vi "test_pid_amplitude.vi"() -> ()   [LabVIEW 2013]
panel:
  out "Waveform Graph 6":dbl[][](graph)
  out "Waveform Graph 5":dbl[](graph)
  in  "Kp":fxp<+/-,32,6>=0.004999995231628418
  in  "Kd/Tau":fxp<+/-,32,6>
  in  "Ki*Tau":fxp<+/-,32,6>=4.999339580535889e-05
  out "Waveform Graph 4":dbl[](graph)
  out "Waveform Graph 3":dbl[](graph)
  out "Waveform Graph 2":dbl[][](graph)
  out "size(s)":i32[](array[numeric])
  out "Waveform Graph":dbl[][](graph)
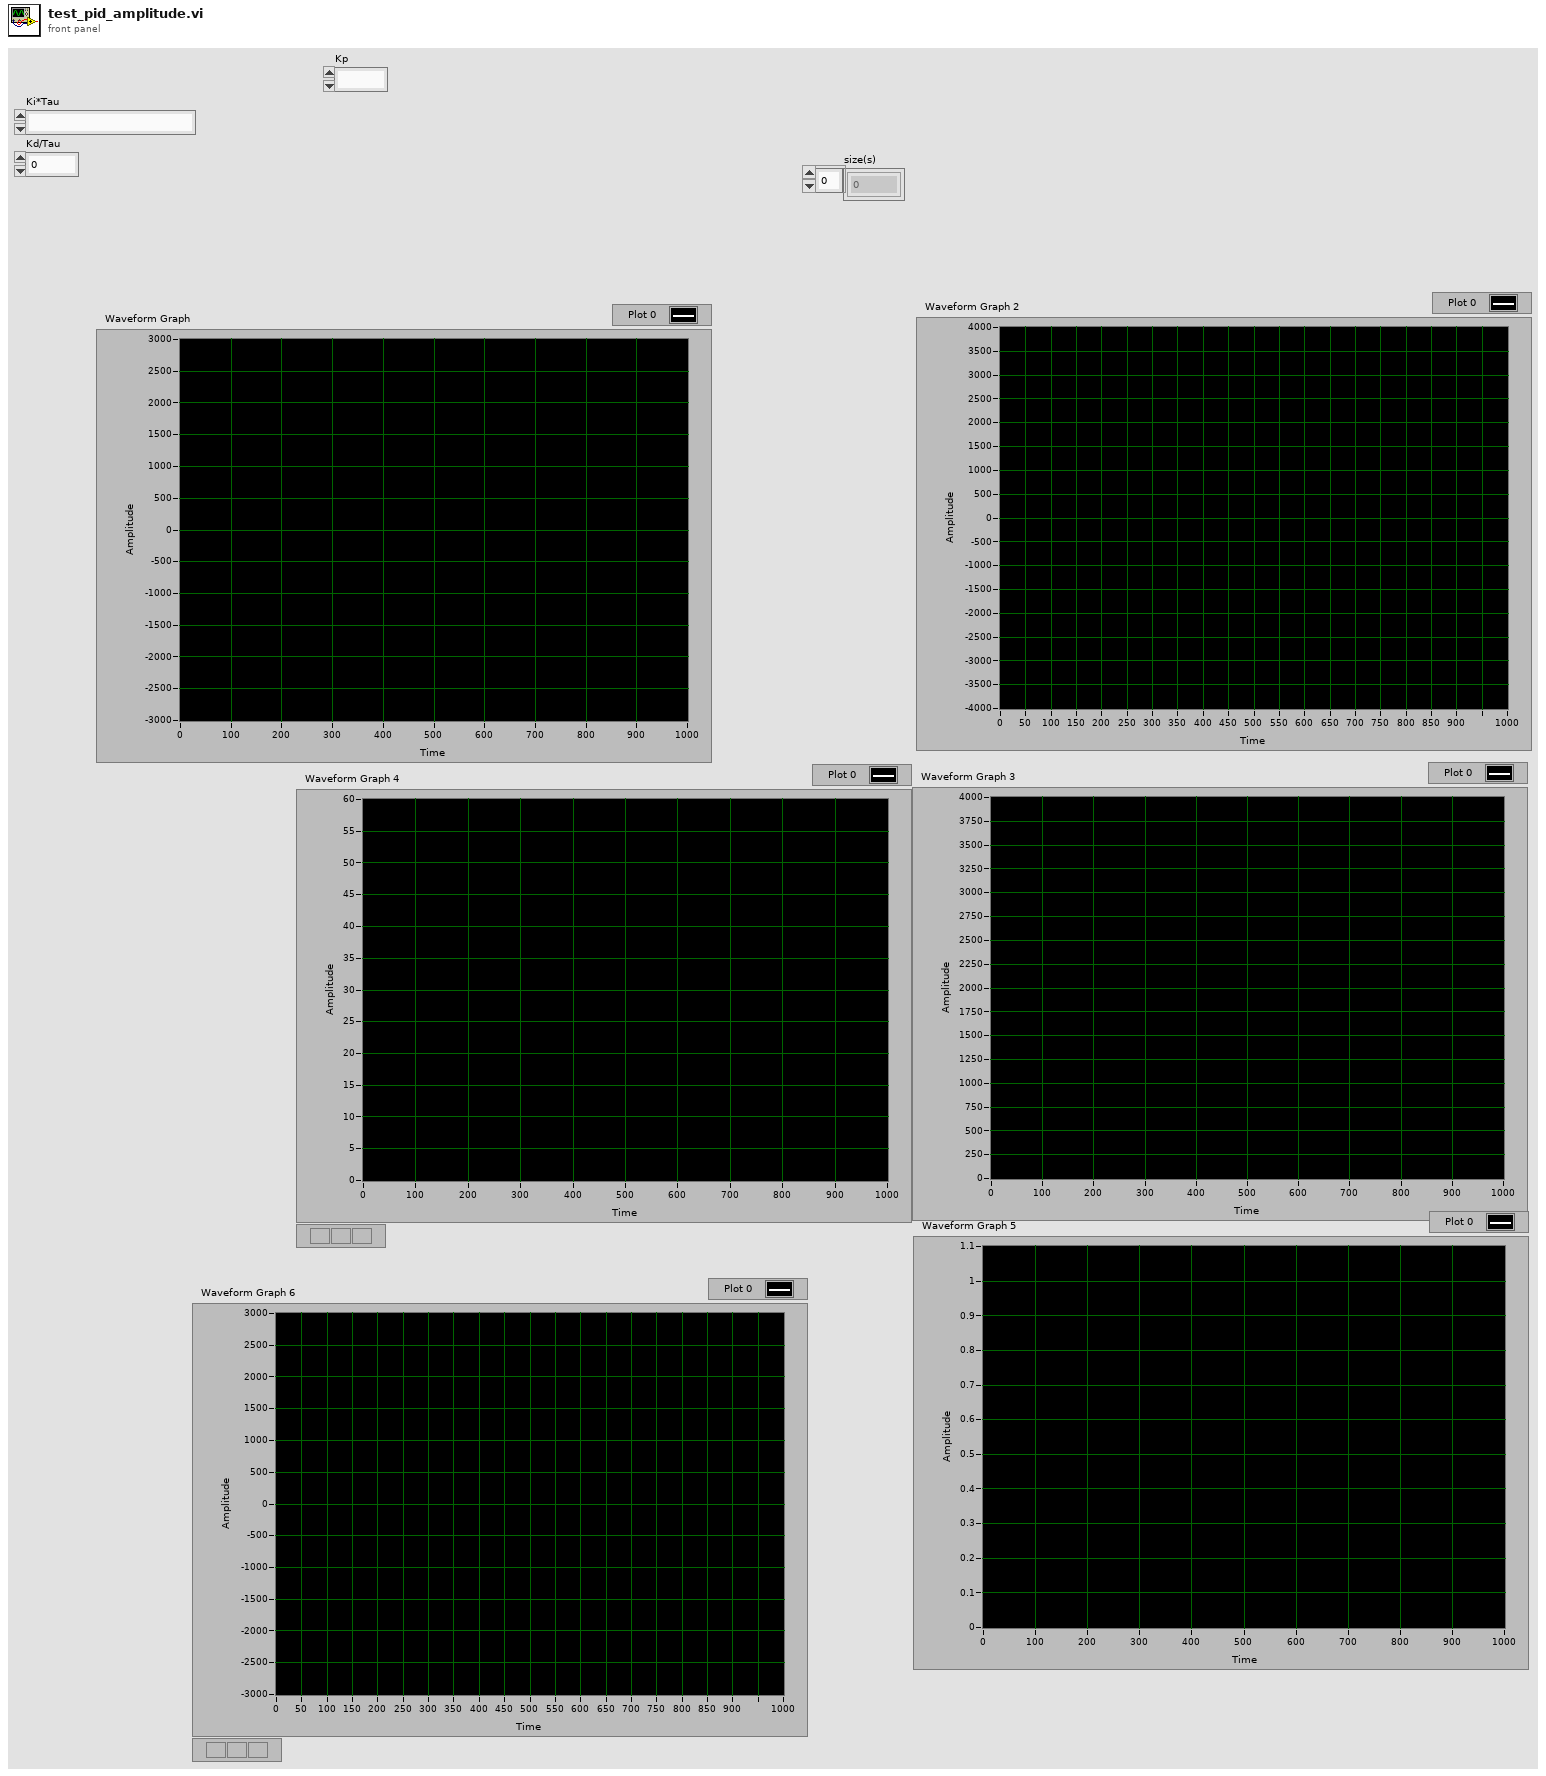
[diagram p1: front panel]
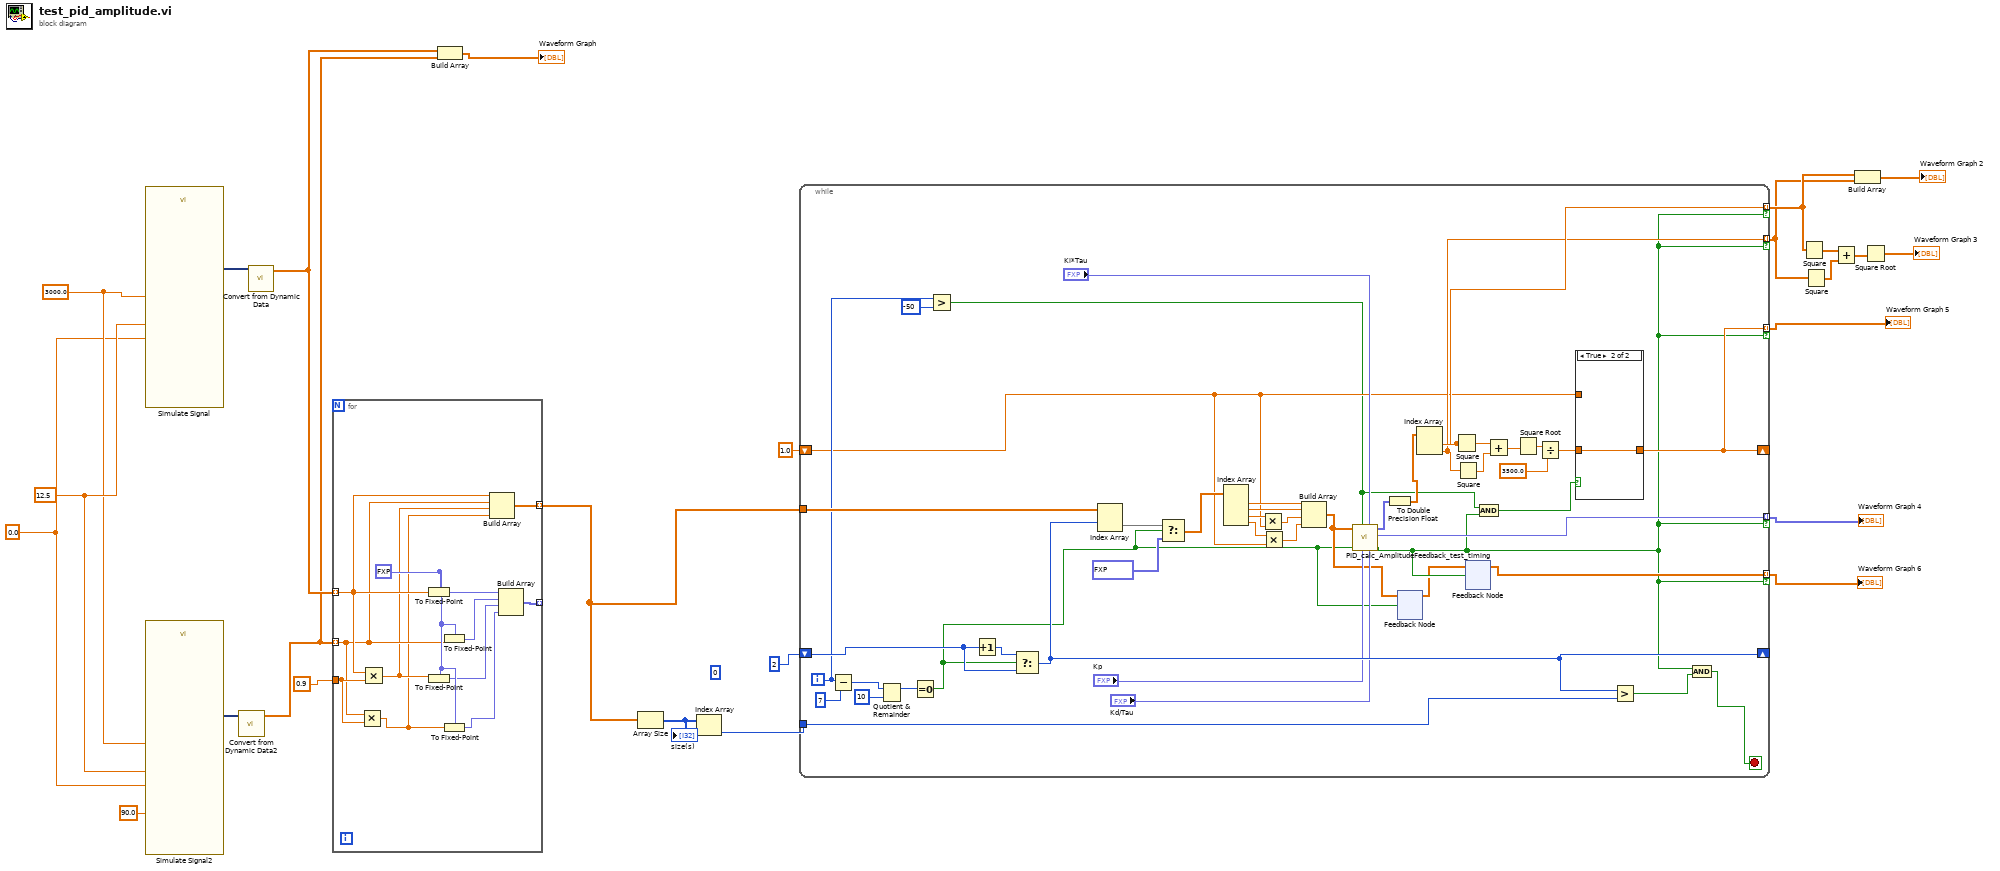
[diagram p0: block diagram]
diagram:
  w12 = 3000.0 ("Amplitude")
  (unwired) 0
  w13 = 12.5 ("Frequency")
  w5 = 0.0 ("Noise amplitude")
  n1 = call "Simulate Signal"("Frequency"=w13, "Amplitude"=w12, "Noise amplitude"=w5) -> ("Sine with Uniform Noise"=w25:dynamicdata)  [unwired: 11 in, 1 out]
  n2 = call "Simulate Signal2"("Frequency"=w13, "Amplitude"=w12, "Phase"=90.0, "Noise amplitude"=w5) -> ("Sine with Uniform Noise"=w23:dynamicdata)  [unwired: 10 in, 1 out]
  n3 = call "Convert from Dynamic Data2"("Dynamic Data Type"=w23) -> ("Array"=w21:dbl[])  [unwired: 3 in]
  n4 = call "Convert from Dynamic Data"("Dynamic Data Type"=w25) -> ("Array"=w22:dbl[])  [unwired: 3 in]
  n5 = for {
    tunnel: w21 -> [w29] mode=indexing
    tunnel: w22 -> [w30] mode=indexing
    tunnel: [w35] -> _ mode=indexing
    tunnel: 0.9 ("y") -> [w34]
    tunnel: [w26] -> w3 mode=indexing
    w33 = fxp<+/-,16,14> 0.0 ("f")
    n6 = Multiply(x=w29, y=w34) -> (x*y=w27:dbl)
    n7 = Multiply(x=w30, y=w34) -> (x*y=w28:dbl)
    n8 = To Fixed-Point(fixed-point type=w33, number=w30) -> (fixed-point=w37:fxp<+/-,16,14>)
    n9 = To Fixed-Point(fixed-point type=w33, number=w28) -> (fixed-point=w31:fxp<+/-,16,14>)
    n10 = To Fixed-Point(fixed-point type=w33, number=w29) -> (fixed-point=w36:fxp<+/-,16,14>)
    n11 = To Fixed-Point(fixed-point type=w33, number=w27) -> (fixed-point=w32:fxp<+/-,16,14>)
    n12 = Build Array(w30, w29, w28, w27) -> (w26:dbl[])
    n13 = Build Array(w37, w36, w31, w32) -> (w35:fxp<+/-,16,14>[])
  }
  n14 = Build Array(w22, w21) -> (→"Waveform Graph":dbl[][])
  n15 = Array Size(array=w3) -> (size(s)=w19:i32[])
  "size(s)" <- w19
  n16 = Index Array(array=w19) -> (element=w17:i32)  [unwired: 1 in]
  n17 = while {
    tunnel: w3 -> [w76]
    shift-right: [w78] -> _
    shift-left: 2 ("y") -> [w79]
    tunnel: [w57] -> w10 mode=indexing if=w41
    tunnel: w17 -> [w70]
    tunnel: [w56] -> w9 mode=indexing if=w41
    tunnel: [w66] -> w6 mode=indexing if=w41
    shift-right: [w45] -> _
    shift-left: 1.0 -> [w46]
    tunnel: [w45] -> w2 mode=indexing if=w41
    tunnel: [w42] -> w1 mode=indexing if=w41
    i -> [w65]
    stop <- w72 stop-if-true
    n18 = Subtract(x=w65, y=7) -> (x-y=w74:i32)
    n19 = Quotient & Remainder(x=w74, y=10) -> (x-y*floor(x/y)=w81:i32)  [unwired: 1 out]
    n20 = Equal To 0?(x=w81) -> (x = 0?=w39:bool)
    n21 = Greater?(x=w65, y=-50) -> (0:w44:bool)
    n22 = Increment(x=w79) -> (x+1=w80:i32)
    n23 = Select(t=w80, s=w39, f=w79) -> (s? t:f=w78:i32)
    n24 = Index Array(array=w76, index (row)=w78) -> (element=w77:dbl[])  [unwired: 1 in]
    n25 = Select(t=w77, s=w39, f=fxp<+/-,16,14>[] [0.0, 0.0, 0.0, 0.0] ("Data in")) -> (s? t:f=w53:dbl[])
    n26 = Index Array(array=w53) -> (element #1=w50:dbl, element #2=w49:dbl, element #3=w52:dbl, element #4=w51:dbl)  [unwired: 4 in]
    n27 = Multiply(x=w52, y=w46) -> (x*y=w48:dbl)
    n28 = Multiply(x=w51, y=w46) -> (x*y=w47:dbl)
    n29 = Build Array(w50, w49, w48, w47) -> (w40:dbl[])
    n30 = call "PID_calc_AmplitudeFeedback_test_timing.vi"("Kd/Tau"="Kd/Tau", "Ki*Tau"="Ki*Tau", "Kp"="Kp", "Enabled"=w44, "input valid"=w39, "Data in"=w40) -> ("output valid"=w41:bool, "c(t)"=w66:fxp<+/-,32,21>, "data out"=w59:fxp<+/-,16,14>[])  [unwired: 2 in, 1 out]
    n31 = To Double Precision Float(number=w59) -> (double precision float=w58:dbl[])
    n32 = feedback #1() -> (w38:dbl[])  [unwired: 1 in]
    n33 = feedback-in #1(w40, w39) -> ()
    n34 = Index Array(array=w58) -> (element #1=w57:dbl, element #2=w56:dbl)  [unwired: 2 in]
    n35 = Square(x=w57) -> (x^2=w63:dbl)
    n36 = Square(x=w56) -> (x^2=w61:dbl)
    n37 = feedback #2() -> (w42:dbl[])  [unwired: 1 in]
    n38 = feedback-in #2(w38, w41) -> ()
    n39 = And(x=w44, y=w41) -> (x .and. y?=w43:bool)
    n40 = Add(x=w63, y=w61) -> (x+y=w62:dbl)
    n41 = Square Root(x=w62) -> (sqrt(x)=w60:dbl)
    n42 = Divide(x=w60, y=3500.0) -> (x/y=w54:dbl)
    n43 = case shown="True" w43 {
      tunnel: w54 -> [_ w84]
      tunnel: [w83 w84] -> w45
      tunnel: w46 -> [w83 _]
      frame False {
      }
      frame True {
      }
    }
    n44 = Greater?(x=w78, y=w70) -> (0:w73:bool)
    n45 = And(x=w41, y=w73) -> (x .and. y?=w72:bool)
  }
  "Waveform Graph 4" <- w6
  "Waveform Graph 5" <- w2
  "Waveform Graph 6" <- w1
  n46 = Square(x=w10) -> (x^2=w14:dbl[])
  n47 = Square(x=w9) -> (x^2=w16:dbl[])
  n48 = Add(x=w14, y=w16) -> (x+y=w15:dbl[])
  n49 = Build Array(w10, w9) -> (→"Waveform Graph 2":dbl[][])
  n50 = Square Root(x=w15) -> (sqrt(x)=→"Waveform Graph 3":dbl[])
